vi "getCapacitance.vi"(8 "error in (no error)":errorcluster, 9 "Channel":i32, 11 "Instrument.CBridge in":refnum<class "Instrument.CBridge.lvclass">) -> (0 "error out":errorcluster, 2 "Capacitance (pF)":dbl, 3 "Instrument.CBridge out":refnum<class "Instrument.CBridge.lvclass">)   [LabVIEW 2019, in "Instrument.CBridge.lvclass"]
uses:
  Instrument.CBridge.lvclass
  Typedefs/CBridge.Commands--Enum.ctl
  e256a054-c19d-4c32-b66d-9d3274a341ad.vi
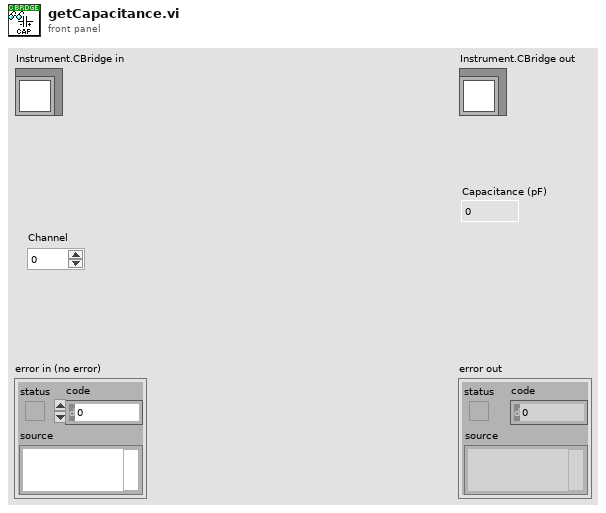
[diagram p1: front panel]
types:
  T1 = typedef "Instrument.CBridge.lvclass/CBridge.Commands--Enum.ctl" = enum16{"getCapacitance"}
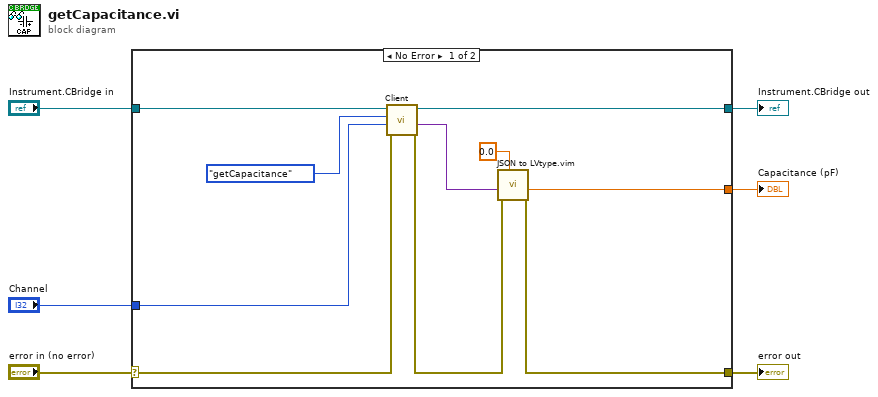
[diagram p0: block diagram]
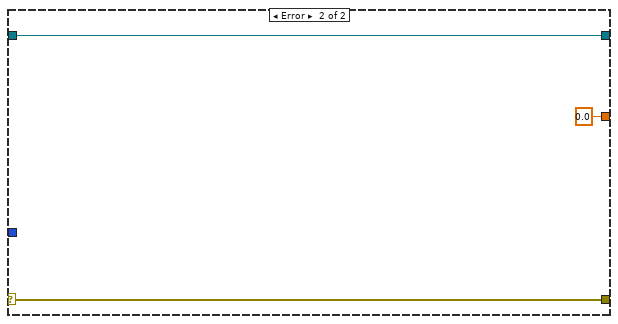
[diagram p2: hidden frame]
diagram:
  n1 = case shown="No Error" "error in (no error)" {
    selector: "error in (no error)" -> [w12 w19]
    tunnel: [w8 w19] -> w5
    tunnel: [w16 w18] -> w3
    tunnel: "Instrument.CBridge in" -> [w13 w18]
    tunnel: [w7 0.0 ("Data out")] -> w2
    tunnel: "Channel" -> [w15 _]
    frame No Error {
      n2 = call-dynamic "Client.vi"("error in (no error)"=w12, "Data in"=w15, "Command in"=CBridge.Commands--Enum."getCapacitance" ("Commands"), "Instrument in"=w13) -> ("error out"=w9:errorcluster, "Data out"=w10:variant, "Instrument out"=w16:refnum<class "Instrument.CBridge.lvclass">)  [unwired: 4 in, 1 out]
      n3 = call "JSON to LVtype.vim"("type"=0.0, "error in (no error)"=w9, "JSON Data in"=w10) -> ("error out"=w8:errorcluster, "Data out"=w7:dbl)  [unwired: 7 in]
    }
    frame Error {
    }
  }
  "error out" <- w5
  "Instrument.CBridge out" <- w3
  "Capacitance (pF)" <- w2
